vi "main.vi"() -> ()   [LabVIEW 2019]
uses:
  THCD_400/thcd_controls/variable_reference.ctl
  Fridge_Valve/cluster_ref_fridge_valve.ctl
  <vilib>/Instr/_visa.llb/VISA Flush IO Buffer Mask.ctl
  <vilib>/Utility/config.llb/Read Key (String).vi
  subvi_main/Global 1.vi
  <vilib>/Utility/config.llb/Read Key (Path).vi
  <vilib>/Instr/_visa.llb/VISA Configure Serial Port (Instr).vi
  <vilib>/Utility/config.llb/Read Key (Double).vi
  <vilib>/Utility/file.llb/Write Delimited Spreadsheet (DBL).vi
  <vilib>/Utility/config.llb/NI_LVConfig.lvlib
panel:
  out "Status":bool
  in  "Fridge Valve Open Sub Panel":bool
  in  "?":bool
  in  "?":bool
  in  "?":bool
  in  "?":bool
  out "Status":bool
  out "FC1":dbl format="%#_13g"
  out "FC2":dbl format="%#_13g"
  out "FM1":dbl format="%#_13g"
  out "Bypass Valve Opening":dbl format="%_3f"
  out "Main\nFlow":dbl
  out "Vacuum Pressure":dbl
  out "He3 Vapor Pressure":dbl
  out "Writing to file":bool
  out "Status":bool
  out "Boolean 2":bool
  in  "stop":bool
  out "Boolean":bool
  out "He4 Pressure":dbl
  out "Backfill\nPressure\n(Torr)":dbl
  in  "?":bool
  out "Run-Valve Opening":dbl format="%_3f"
  out "Nose Level (%)":dbl(slide) scale=0.0..100.0
  out "?":u8(slide) scale=0.0..100.0
  in  "?":bool
  out "Sep. Pressure":dbl
  out "?":dbl
  in  "kill process":bool
  out "Array 2":bool[](array[boolean])
  out "Error at VISA Read 7":errorcluster
  out "Error at segmenting output 6":errorcluster
  out "Array":bool[](array[boolean])
  out "Error at segmenting output 5":errorcluster
  out "Error at VISA Read 6":errorcluster
  in  "Numeric":dbl
  out "read buffer":string
  in  "STOP VI":bool
  in  "stop 2":bool
  out "error out 5":errorcluster
  out "error out 4":errorcluster
  out "error out 3":errorcluster
  out "error out 2":errorcluster
  out "value 2":path
  out "value":path
  out "error out":errorcluster
  # "CryoControls"
  # "Torr"
  # "Magnet Flow"
  # "Seperator Flow"
  # "Backfill Pressure (Torr)"
  # "Torr"
  # "n/a"
  # "Torr"
  # "MKS 670 / 1000"
  # "MKS 670 /   100"
  # "MKS 670 / He3"
  # "MKS 946"
  # "THCD-400"
  # "%"
  # "%"
  # "Torr"
  # "Fridge Valve"
  # "Fridge Flow"
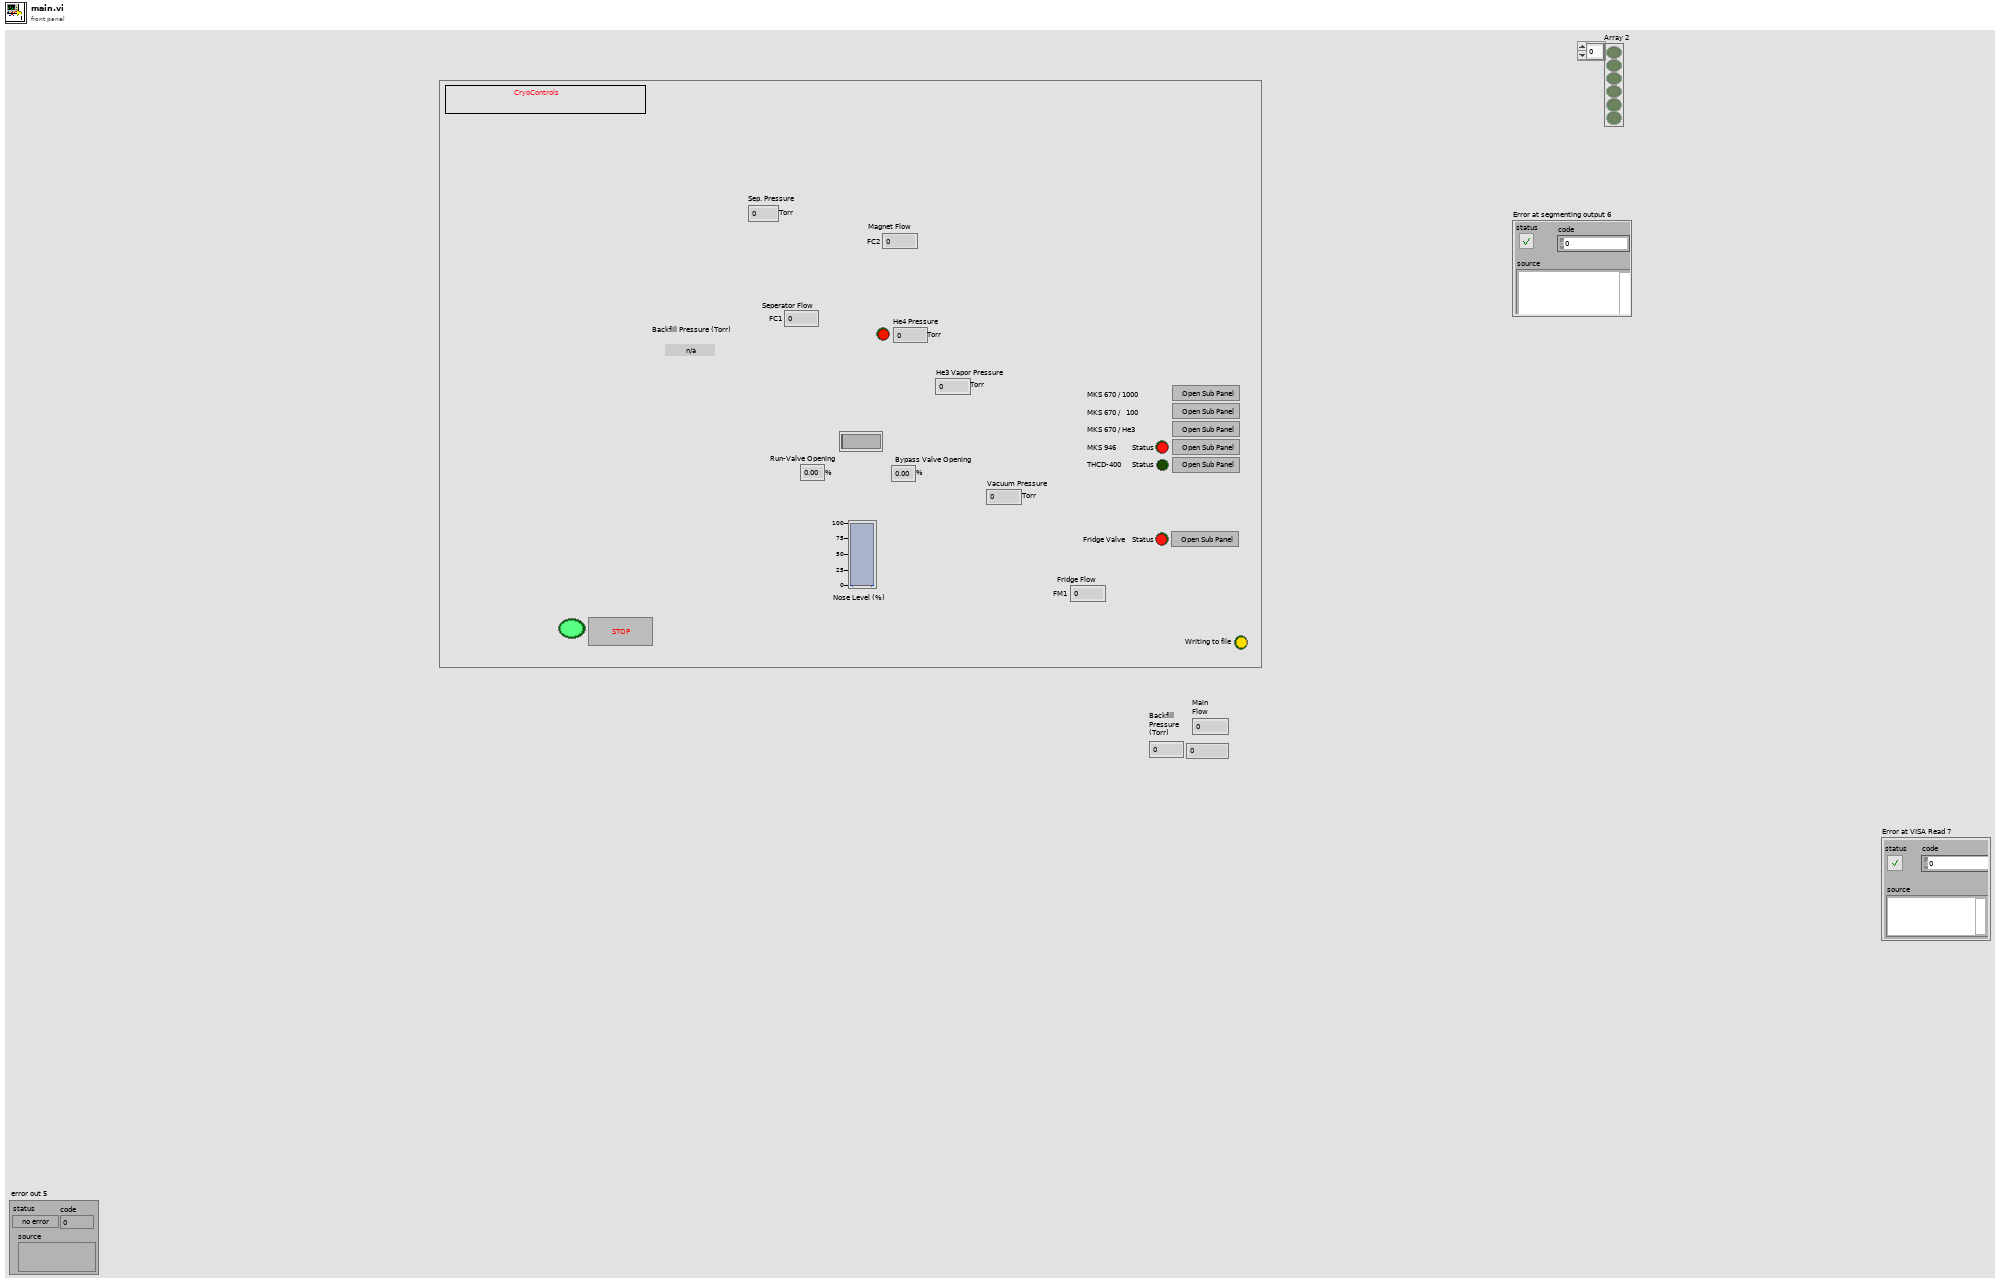
[diagram p1: front panel]
types:
  T1 = typedef "cluster_ref_fridge_valve.ctl" = cluster{"Status":refnum<vi>, "RVO":refnum<vi>, "BVO":refnum<vi>, "He Level":refnum<vi>}
  T2 = typedef "variable_reference.ctl" = cluster{"Status":refnum<vi>, "FM1":refnum<vi>, "FC1":refnum<vi>, "FC2":refnum<vi>}
  T3 = typedef "NI_LVConfig.lvlib/Config Data RefNum.ctl" = refnum<k1>
  T4 = typedef "VISA Flush IO Buffer Mask.ctl" = u16
  T5 = typedef "Semaphore RefNum" = refnum<k1>
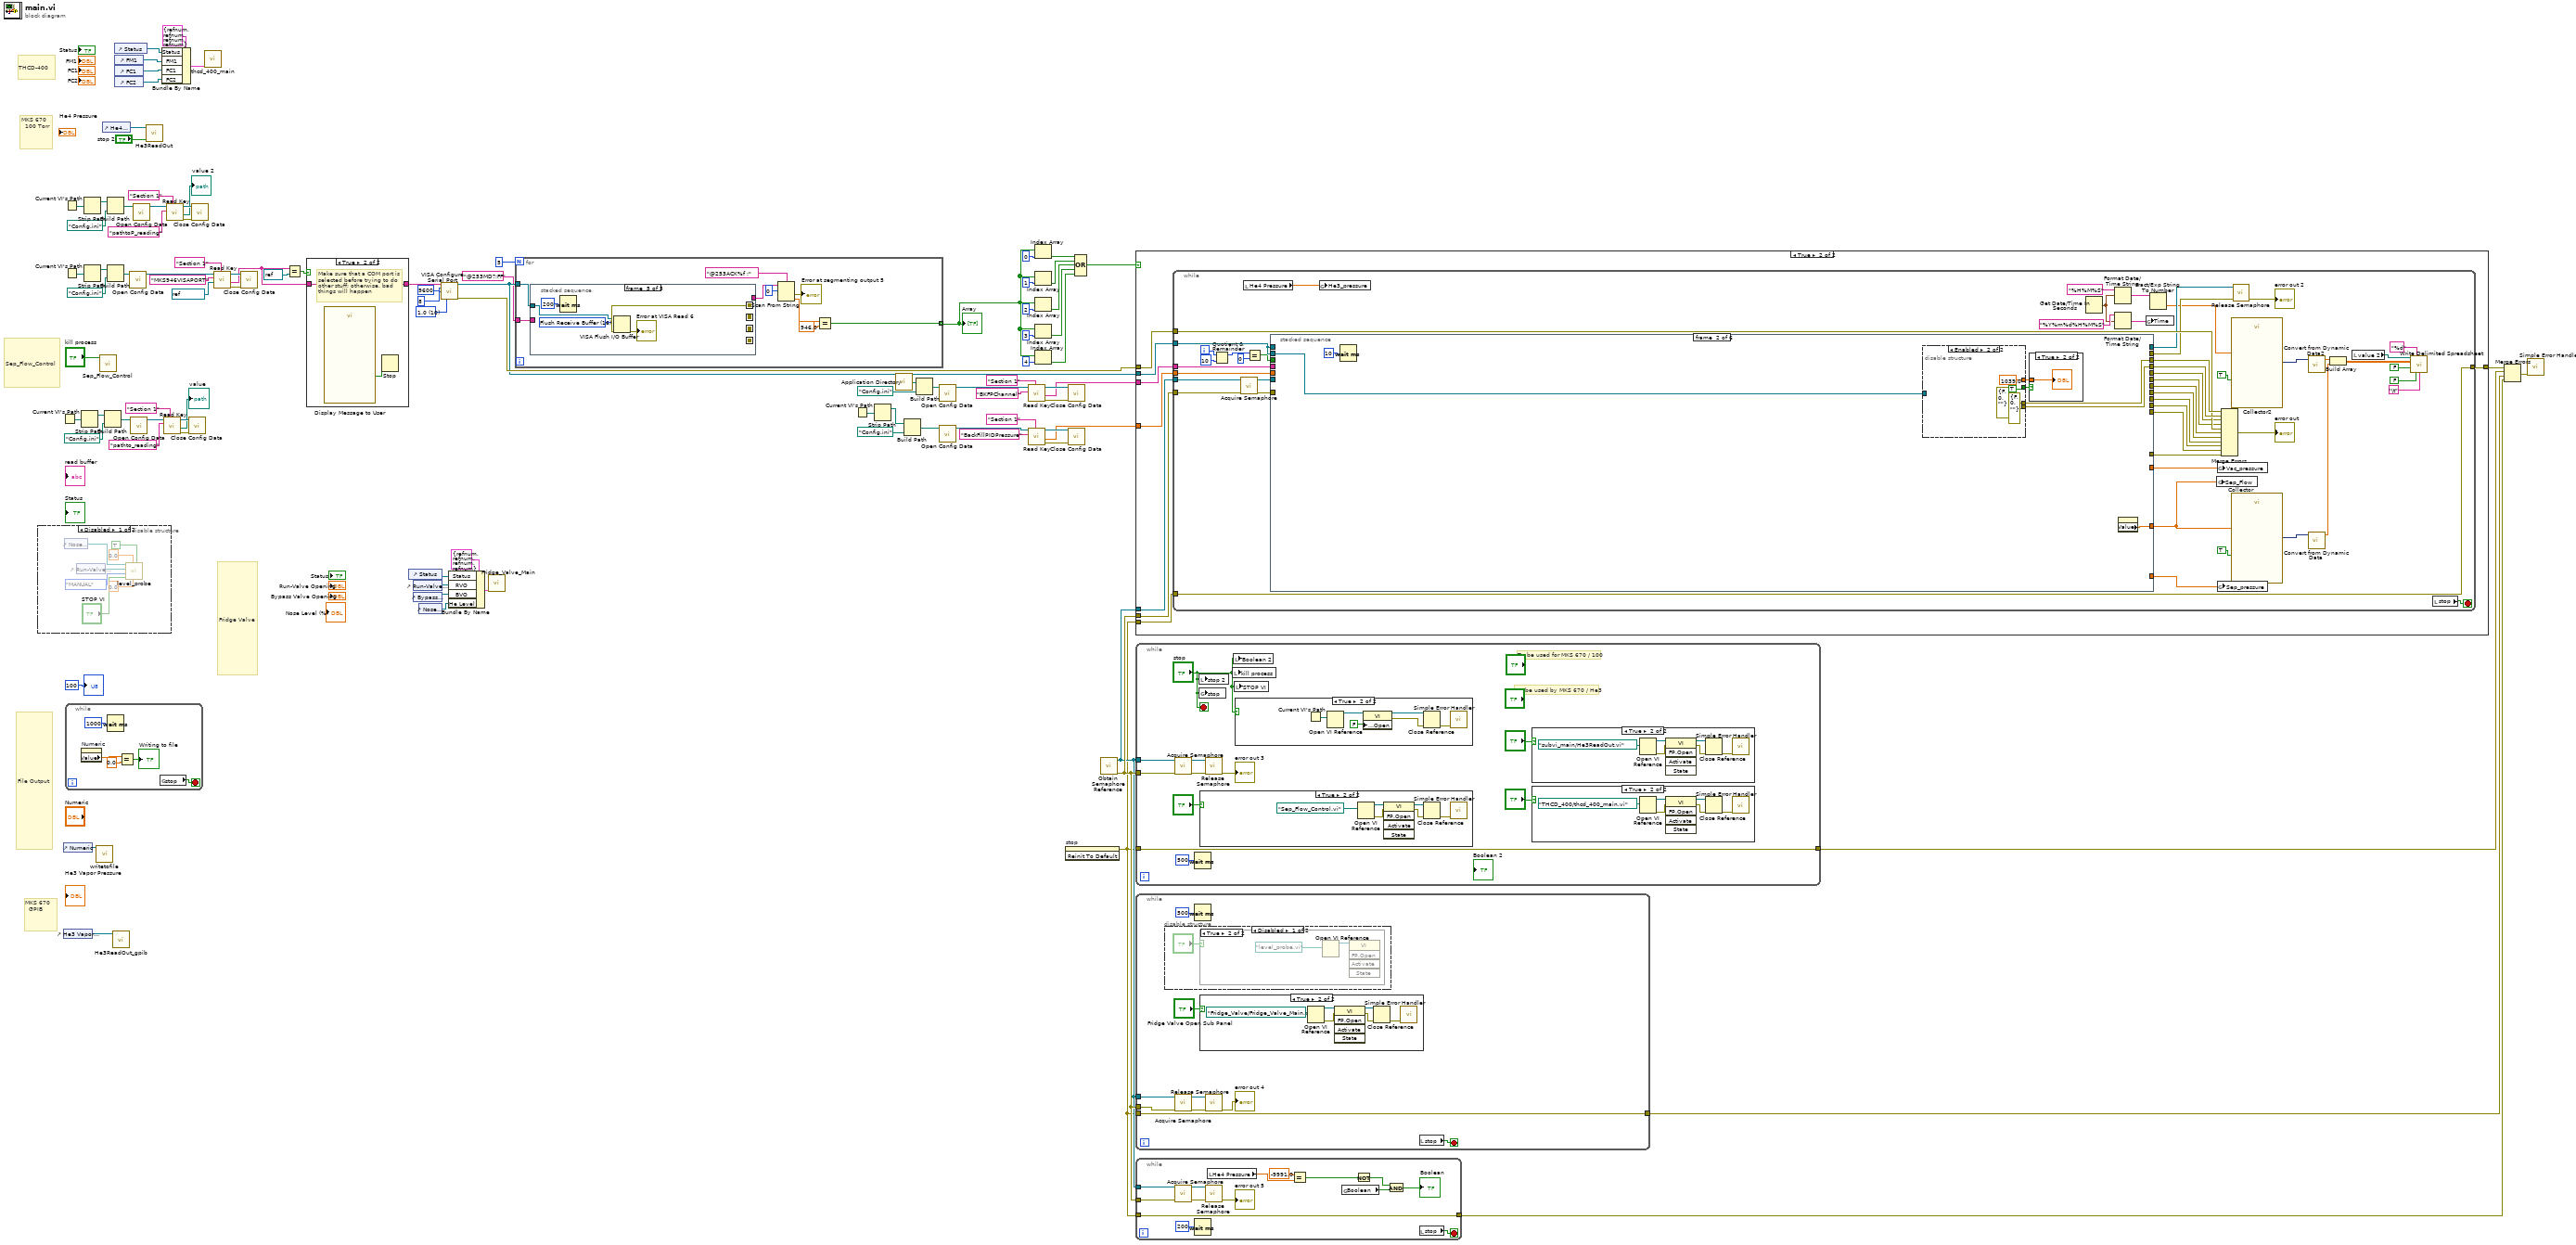
[diagram p0: block diagram]
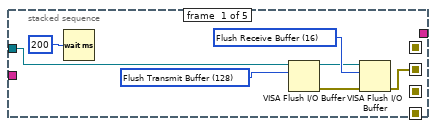
[diagram p3: hidden frame]
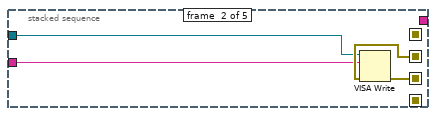
[diagram p4: hidden frame]
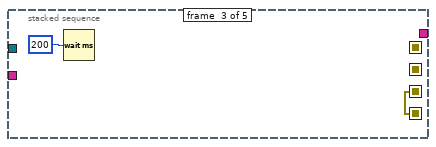
[diagram p5: hidden frame]
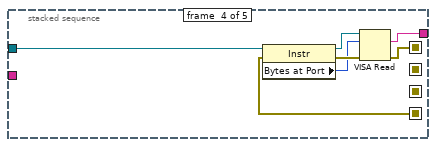
[diagram p6: hidden frame]
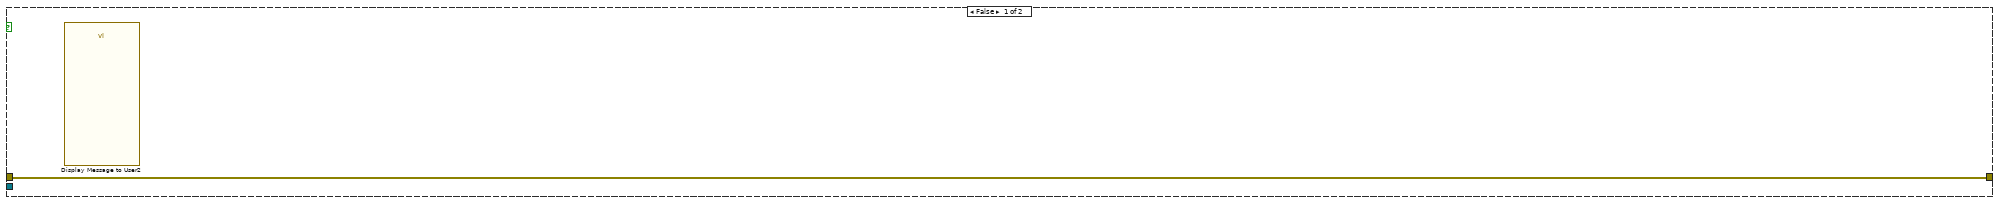
[diagram p7: hidden frame]
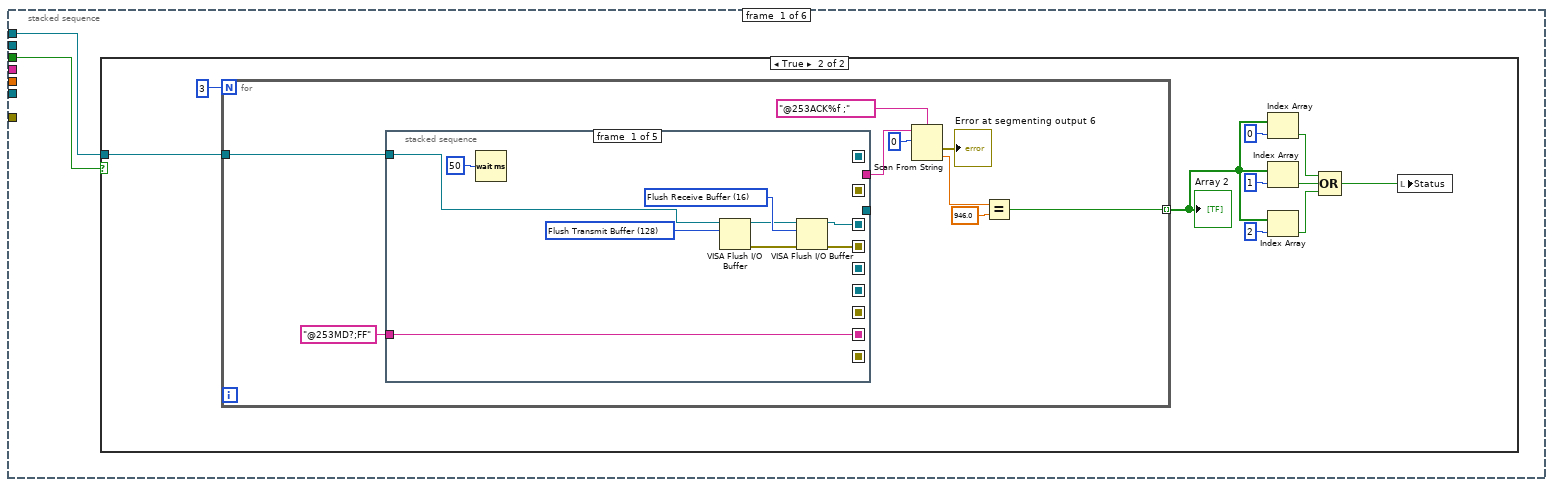
[diagram p8: hidden frame]
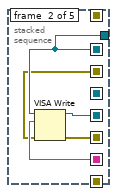
[diagram p10: hidden frame]
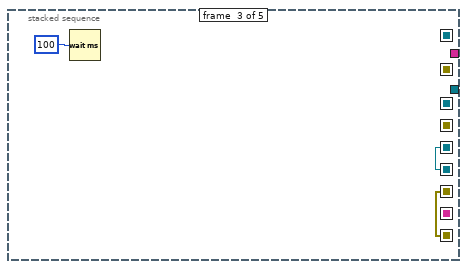
[diagram p11: hidden frame]
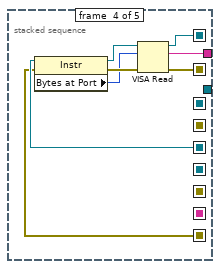
[diagram p12: hidden frame]
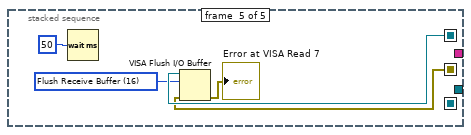
[diagram p13: hidden frame]
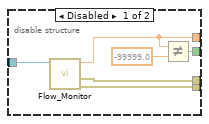
[diagram p14: hidden frame]
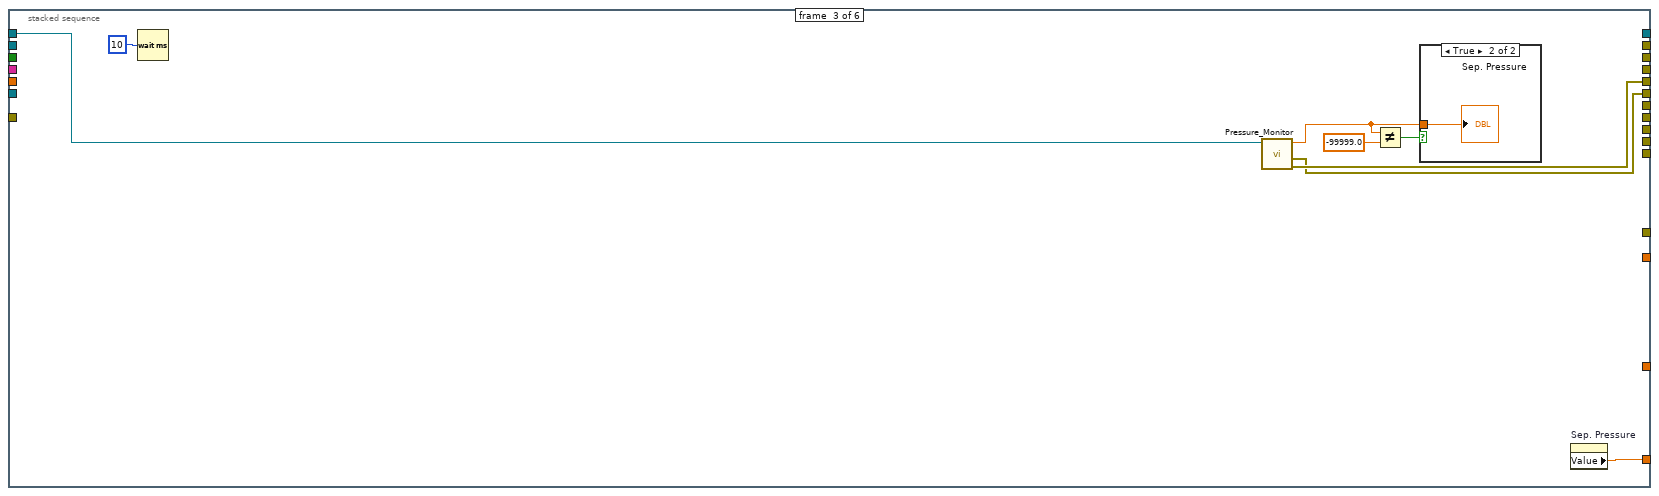
[diagram p16: hidden frame]
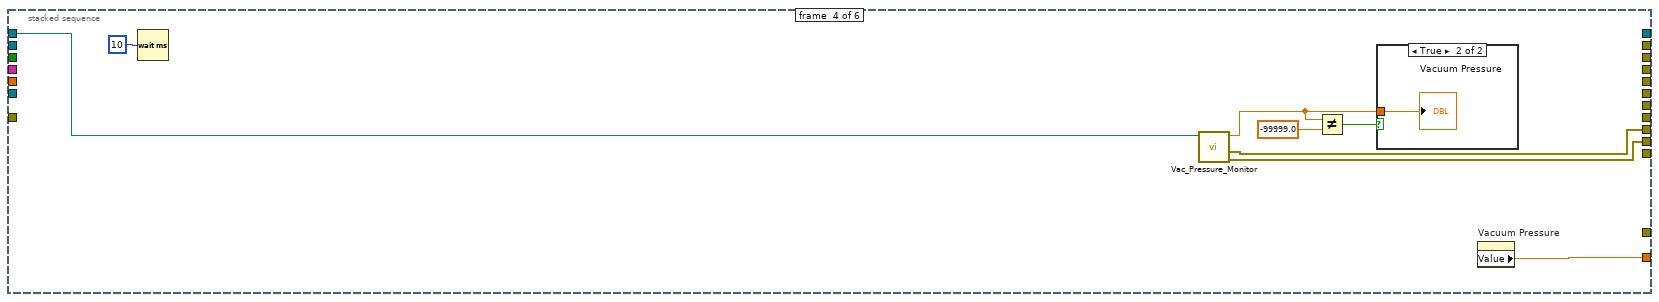
[diagram p18: hidden frame]
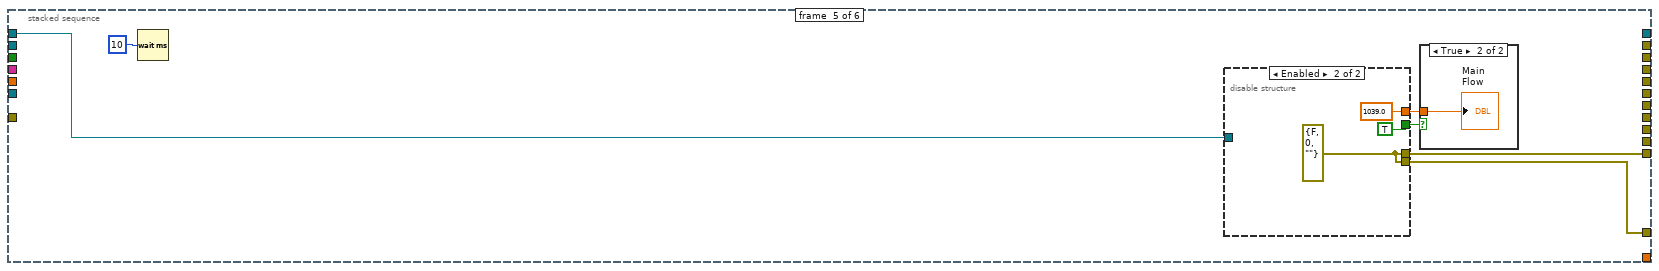
[diagram p20: hidden frame]
diagram:
  w93 = u16 10 items=["1.0"=10, "1.5"=15, "2.0"=20] ("stop bits (10: 1 bit)")
  # "Sep_Flow_Control"
  # "Fridge Valve"
  # "File Output"
  # "MKS 670  \n  GPIB"
  # "MKS 670  \n  100 Torr"
  # "THCD-400"
  n1 = disable-structure shown="Disabled" {
    frame Disabled {
      n2 = control-ref of="Nose Level (%)"() -> (w104:refnum<vi>)
      n3 = control-ref of="Run-Valve Opening"() -> (w105:refnum<vi>)
      n4 = call "level_probe.vi"("Run VI"=TRUE, "Set # of Turns Open (Man)"=0.0, "Target Level (Auto)"=0.0, "stop"="STOP VI", "Mode"=enum32{"AUTOMATIC", "MANUAL"}."MANUAL", "position"=w105, "level"=w104) -> ()  [unwired: 5 in]
    }
    frame Enabled {
    }
  }
  n5 = Current VI's Path() -> (path=w26:path)
  n6 = control-ref of="Numeric"() -> (w46:refnum<vi>)
  n7 = control-ref of="He3 Vapor Pressure"() -> (w14:refnum<vi>)
  n8 = Current VI's Path() -> (path=w30:path)
  n9 = Current VI's Path() -> (path=w28:path)
  n10 = while {
    stop <- w107 stop-if-true
    n11 = property on="Numeric" class="DigNum (strict)"() -> ("Value"=w109:dbl)  [unwired: 2 in, 2 out]
    n12 = Wait (ms)(milliseconds to wait=u32 1000) -> ()  [unwired: 1 out]
    n13 = Equal?(x=w109, y=0.0) -> (x = y?=→"Writing to file":bool)
    n14 = global read "Global 1.vi" "stop"() -> (w107:bool)
  }
  n15 = Strip Path(path=w26) -> (stripped path=w25:path)  [unwired: 1 out]
  n16 = Strip Path(path=w30) -> (stripped path=w29:path)  [unwired: 1 out]
  n17 = Strip Path(path=w28) -> (stripped path=w27:path)  [unwired: 1 out]
  n18 = call "writetofile.vi"("reference"=w46) -> ()  [unwired: 9 in]
  n19 = call "Sep_Flow_Control.vi"("kill process"="kill process") -> ()  [unwired: 11 in]
  n20 = control-ref of="He4 Pressure"() -> (w56:refnum<vi>)
  n21 = Build Path(base path=w25, name or relative path=path "Config.ini" ("default name")) -> (appended path=w67:path)
  n22 = Build Path(base path=w29, name or relative path=path "Config.ini" ("default name")) -> (appended path=w80:path)
  n23 = Build Path(base path=w27, name or relative path=path "Config.ini" ("default name")) -> (appended path=w86:path)
  n24 = call "He3ReadOut_gpib.vi"("reference"=w14) -> ()  [unwired: 11 in]
  n25 = control-ref of="Status"() -> (w11:refnum<vi>)
  n26 = control-ref of="FM1"() -> (w10:refnum<vi>)
  n27 = control-ref of="FC1"() -> (w9:refnum<vi>)
  n28 = control-ref of="FC2"() -> (w8:refnum<vi>)
  n29 = call <vilib>:"Open Config Data.vi"("configuration file path"=w86) -> ("refnum"=w91:T3)  [unwired: 8 in, 2 out]
  n30 = call <vilib>:"Open Config Data.vi"("configuration file path"=w67) -> ("refnum"=w66:T3)  [unwired: 8 in, 2 out]
  n31 = call <vilib>:"Open Config Data.vi"("configuration file path"=w80) -> ("refnum"=w69:T3)  [unwired: 8 in, 2 out]
  n32 = call "He3ReadOut.vi"("reference"=w56, "stop"="stop 2") -> ()  [unwired: 7 in]
  n33 = Bundle By Name(cluster=T2 {"Status"=refnum, "FM1"=refnum, "FC1"=refnum, "FC2"=refnum} ("variable_ref"), "Status"=w11, "FM1"=w10, "FC1"=w9, "FC2"=w8) -> (w7:T2)
  n34 = call-poly <vilib>:"Read Key.vi"("section"="Section 1", "key"="pathto_reading", "refnum"=w66) -> ("error out"=w76:errorcluster, "value"=→"value":path, "refnum out"=w78:T3)  [unwired: 5 in, 1 out]
  n35 = call-poly <vilib>:"Read Key.vi"("section"="Section 1", "key"="pathtoP_reading", "refnum"=w69) -> ("error out"=w71:errorcluster, "value"=→"value 2":path, "refnum out"=w73:T3)  [unwired: 5 in, 1 out]
  n36 = call <vilib>:"Close Config Data.vi"("error in (no error)"=w76, "refnum"=w78) -> ()  [unwired: 8 in, 2 out]
  n37 = call <vilib>:"Close Config Data.vi"("error in (no error)"=w71, "refnum"=w73) -> ()  [unwired: 8 in, 2 out]
  n38 = call "thcd_400_main.vi"("variable_ref"=w7) -> ()  [unwired: 10 in]
  n39 = call-poly <vilib>:"Read Key.vi"("section"="Section 1", "default value"=refnum<visa-resource-name> "COM5" ("VISA resource name"), "key"="MKS946VISAPORT", "refnum"=w91) -> ("error out"=w85:errorcluster, "value"=w83:string, "refnum out"=w89:T3)  [unwired: 4 in, 1 out]
  n40 = call <vilib>:"Close Config Data.vi"("error in (no error)"=w85, "refnum"=w89) -> ()  [unwired: 8 in, 2 out]
  n41 = Equal?(x=w83, y=refnum<visa-resource-name> refnum) -> (x = y?=w97:bool)
  n42 = case shown="True" w97 {
    tunnel: [w111 w112] -> w98
    tunnel: w83 -> [w111 w112]
    frame False {
    }
    frame True {
      # "Make sure that a COM port is\nselected before trying to do\nother stuff; otherwise, bad\nthings will happen"
      n43 = call "Display Message to User"() -> ("Got it, thanks"=w113:bool)  [unwired: 10 in, 1 out]
      n44 = Stop(stop? (T)=w113) -> ()
    }
  }
  n45 = control-ref of="Status"() -> (w6:refnum<vi>)
  n46 = control-ref of="Run-Valve Opening"() -> (w4:refnum<vi>)
  n47 = control-ref of="Bypass Valve Opening"() -> (w3:refnum<vi>)
  n48 = control-ref of="Nose Level (%)"() -> (w1:refnum<vi>)
  n49 = call-poly "VISA Configure Serial Port"("VISA resource name"=w98, "baud rate (9600)"=u32 9600, "data bits (8)"=u16 8, "stop bits (10: 1 bit)"=w93) -> ("VISA resource name out"=w45:refnum<visa-resource-name>, "error out"=w92:errorcluster)  [unwired: 10 in]
  n50 = Bundle By Name(cluster=T1 {"Status"=refnum, "RVO"=refnum, "BVO"=refnum, "He Level"=refnum} ("input cluster"), "Status"=w6, "RVO"=w4, "BVO"=w3, "He Level"=w1) -> (w2:T1)
  n51 = call "Fridge_Valve_Main.vi"("cluster_ref_fridge_valve"=w2) -> ()  [unwired: 11 in]
  n52 = for {
    N: 5 -> [_]
    tunnel: w45 -> [w116]
    tunnel: "@253MD?;FF" ("string") -> [w115]
    tunnel: [w114] -> w31 mode=indexing
    n53 = stacked-sequence {
      seq-local: [w124 _ _ _ _] -> [_ w132 _ _ _]
      seq-local: [_ w133 _ _ _] -> [_ _ w134 _ _]
      seq-local: [_ _ w134 _ _] -> [_ _ _ w139 _]
      seq-local: [_ _ _ w138 _] -> [_ _ _ _ w146]
      tunnel: w115 -> [_ w130 _ _ _]
      tunnel: w116 -> [w125 w131 _ w136 w143]
      tunnel: [_ _ _ w137 _] -> w117
      frame #0 {
        w129 = T4 16 items=["Flush Receive Buffer"=16, "Write Transmit Buffer to Device"=32, "Flush Receive Buffer (No I/O)"=64, "Flush Transmit Buffer"=128] ("Mask")
        w126 = T4 128 items=["Flush Receive Buffer"=16, "Write Transmit Buffer to Device"=32, "Flush Receive Buffer (No I/O)"=64, "Flush Transmit Buffer"=128] ("Mask")
        n54 = Wait (ms)(milliseconds to wait=u32 200) -> ()  [unwired: 1 out]
        n55 = VISA Flush I/O Buffer(VISA resource name=w125, mask (16)=w126) -> (VISA resource name out=w127:refnum<visa-resource-name>, error out=w128:errorcluster)  [unwired: 1 in]
        n56 = VISA Flush I/O Buffer(VISA resource name=w127, mask (16)=w129, error in (no error)=w128) -> (error out=w124:errorcluster)  [unwired: 1 out]
      }
      frame #1 {
        n57 = VISA Write(VISA resource name=w131, write buffer=w130, error in (no error)=w132) -> (error out=w133:errorcluster)  [unwired: 2 out]
      }
      frame #2 {
        n58 = Wait (ms)(milliseconds to wait=u32 200) -> ()  [unwired: 1 out]
      }
      frame #3 {
        n59 = property class="Instr"(reference=w136, error in=w139) -> (reference out=w140:refnum<visa-resource-name>, error out=w142:errorcluster, "Bytes at Port"=w141:u32)
        n60 = VISA Read(VISA resource name=w140, byte count=w141, error in (no error)=w142) -> (read buffer=w137:string, error out=w138:errorcluster)  [unwired: 2 out]
      }
      frame #4 {
        w144 = T4 16 items=["Flush Receive Buffer"=16, "Write Transmit Buffer to Device"=32, "Flush Receive Buffer (No I/O)"=64, "Flush Transmit Buffer"=128] ("Mask")
        n61 = Wait (ms)(milliseconds to wait=u32 200) -> ()  [unwired: 1 out]
        n62 = VISA Flush I/O Buffer(VISA resource name=w143, mask (16)=w144, error in (no error)=w146) -> (error out=→"Error at VISA Read 6":errorcluster)  [unwired: 1 out]
      }
    }
    n63 = Scan From String(format string="@253ACK%f ;", input string=w117, initial scan location=u32 0) -> (error out=→"Error at segmenting output 5":errorcluster, output 1=w119:dbl)  [unwired: 2 in, 2 out]
    n64 = Equal?(x=w119, y=946.0) -> (x = y?=w114:bool)
  }
  "Array" <- w31
  n65 = Current VI's Path() -> (path=w17:path)
  n66 = Strip Path(path=w17) -> (stripped path=w16:path)  [unwired: 1 out]
  n67 = call <vilib>:"Application Directory.vi"() -> ("Application Directory"=w58:path)
  n68 = Build Path(base path=w16, name or relative path=path "Config.ini" ("default name")) -> (appended path=w19:path)
  n69 = Build Path(base path=w58, name or relative path=path "Config.ini" ("default name")) -> (appended path=w60:path)
  n70 = call <vilib>:"Open Config Data.vi"("configuration file path"=w60) -> ("refnum"=w65:T3)  [unwired: 8 in, 2 out]
  n71 = call <vilib>:"Open Config Data.vi"("configuration file path"=w19) -> ("refnum"=w24:T3)  [unwired: 8 in, 2 out]
  n72 = call-poly <vilib>:"Read Key.vi"("section"="Section 1", "key"="BKFPChannel", "refnum"=w65) -> ("error out"=w59:errorcluster, "value"=w57:string, "refnum out"=w63:T3)  [unwired: 5 in, 1 out]
  n73 = call-poly <vilib>:"Read Key.vi"("section"="Section 1", "key"="BackFillPIDPressure", "refnum"=w24) -> ("error out"=w18:errorcluster, "value"=w15:dbl, "refnum out"=w22:T3)  [unwired: 5 in, 1 out]
  n74 = Index Array(array=w31, index=0) -> (element=w36:bool)
  n75 = Index Array(array=w31, index=1) -> (element=w37:bool)
  n76 = Index Array(array=w31, index=2) -> (element=w35:bool)
  n77 = Index Array(array=w31, index=3) -> (element=w34:bool)
  n78 = Index Array(array=w31, index=4) -> (element=w33:bool)
  n79 = invoke on="stop" class="Bool (strict)" method="Reinit To Default"() -> (error out=w49:errorcluster)  [unwired: 3 in, 2 out]
  n80 = call <vilib>:"Close Config Data.vi"("error in (no error)"=w59, "refnum"=w63) -> ()  [unwired: 8 in, 2 out]
  n81 = call <vilib>:"Close Config Data.vi"("error in (no error)"=w18, "refnum"=w22) -> ()  [unwired: 8 in, 2 out]
  n82 = Compound Arithmetic op=OR(w36, w37, w35, w34, w33) -> (w32:bool)
  n83 = call <vilib>:"Obtain Semaphore Reference.vi"() -> ("error out"=w51:errorcluster, "semaphore"=w50:T5)  [unwired: 5 in, 1 out]
  n84 = case shown="True" w32 {
    tunnel: w92 -> [w148 w156]
    tunnel: w57 -> [_ w155]
    tunnel: [w148 w150] -> w55
    tunnel: w51 -> [_ w154]
    tunnel: w50 -> [_ w153]
    tunnel: w49 -> [_ w152]
    tunnel: w45 -> [_ w151]
    tunnel: w15 -> [_ w149]
    frame False {
      n85 = call "Display Message to User2"() -> ()  [unwired: 10 in, 2 out]
    }
    frame True {
      n86 = while {
        tunnel: w151 -> [w190]
        tunnel: w156 -> [w189]
        tunnel: w155 -> [w185]
        tunnel: w153 -> [w182]
        tunnel: w154 -> [w181]
        tunnel: w152 -> [w175]
        tunnel: [w175] -> w150
        tunnel: w149 -> [w163]
        i -> [w173]
        stop <- w174 stop-if-true
        n87 = Quotient & Remainder(x=w173, y=10) -> (x-y*floor(x/y)=w171:i32)  [unwired: 1 out]
        n88 = call <vilib>:"Acquire Semaphore.vi"("error in (no error)"=w181, "semaphore"=w182) -> ("error out"=w179:errorcluster, "semaphore out"=w180:T5)  [unwired: 3 in, 1 out]
        n89 = local read "He4 Pressure"() -> (w166:dbl)
        n90 = Equal?(x=w171, y=0) -> (x = y?=w169:bool)
        n91 = stacked-sequence {
          tunnel: w190 -> [_ w262 _ _ _ _]
          tunnel: w190 -> [w209 _ w280 w289 w297 w314]
          tunnel: w180 -> [_ _ _ _ _ w313]
          tunnel: w179 -> [_ _ _ _ _ w311]
          tunnel: w169 -> [w208 _ _ _ _ _]
          tunnel: w185 -> [_ _ _ _ _ w315]
          tunnel: w163 -> [_ _ _ _ _ w312]
          tunnel: [_ w259 _ _ _ _] -> w207
          tunnel: [_ w260 _ _ _ _] -> w206
          tunnel: [_ w261 _ _ _ _] -> w167
          tunnel: [_ _ w279 _ _ _] -> w164
          tunnel: [_ _ w278 _ _ _] -> w184
          tunnel: [_ _ w277 _ _ _] -> w183
          tunnel: [_ _ _ w288 _ _] -> w161
          tunnel: [_ _ _ w287 _ _] -> w160
          tunnel: [_ _ _ w286 _ _] -> w159
          tunnel: [_ _ _ _ _ w321] -> w187
          tunnel: [_ _ _ _ _ w320] -> w186
          tunnel: [_ _ _ _ _ w313] -> w178
          tunnel: [_ _ _ _ _ w311] -> w177
          tunnel: [_ _ _ _ w296 _] -> w158
          tunnel: [_ _ _ _ w295 _] -> w157
          frame #0 {
            n92 = case shown="True" w208 {
              tunnel: w209 -> [_ w210]
              frame False {
              }
              frame True {
                n93 = for {
                  N: 3 -> [_]
                  tunnel: w210 -> [w222]
                  tunnel: [w221] -> w219 mode=indexing
                  n94 = stacked-sequence {
                    seq-local: [w237 _ _ _ _] -> [_ w242 _ _ _]
                    seq-local: [w231 _ _ _ _] -> [_ w239 _ _ _]
                    seq-local: [w230 _ _ _ _] -> [_ w238 _ _ _]
                    seq-local: [_ w241 _ _ _] -> [_ _ w244 _ _]
                    seq-local: [_ w240 _ _ _] -> [_ _ w243 _ _]
                    seq-local: [_ _ w244 _ _] -> [_ _ _ w250 _]
                    seq-local: [_ _ w243 _ _] -> [_ _ _ w249 _]
                    seq-local: [_ _ _ w248 _] -> [_ _ _ _ w257]
                    seq-local: [_ _ _ w247 _] -> [_ _ _ _ w256]
                    tunnel: "@253MD?;FF" ("string") -> [w237 _ _ _ _]
                    tunnel: w222 -> [w232 _ _ _ _]
                    tunnel: [_ w239 _ _ _] -> _
                    tunnel: [_ _ _ w246 _] -> w223
                    frame #0 {
                      w236 = T4 16 items=["Flush Receive Buffer"=16, "Write Transmit Buffer to Device"=32, "Flush Receive Buffer (No I/O)"=64, "Flush Transmit Buffer"=128] ("Mask")
                      w233 = T4 128 items=["Flush Receive Buffer"=16, "Write Transmit Buffer to Device"=32, "Flush Receive Buffer (No I/O)"=64, "Flush Transmit Buffer"=128] ("Mask")
                      n95 = Wait (ms)(milliseconds to wait=u32 50) -> ()  [unwired: 1 out]
                      n96 = VISA Flush I/O Buffer(VISA resource name=w232, mask (16)=w233) -> (VISA resource name out=w234:refnum<visa-resource-name>, error out=w235:errorcluster)  [unwired: 1 in]
                      n97 = VISA Flush I/O Buffer(VISA resource name=w234, mask (16)=w236, error in (no error)=w235) -> (VISA resource name out=w231:refnum<visa-resource-name>, error out=w230:errorcluster)
                    }
                    frame #1 {
                      n98 = VISA Write(VISA resource name=w239, write buffer=w242, error in (no error)=w238) -> (VISA resource name out=w241:refnum<visa-resource-name>, error out=w240:errorcluster)  [unwired: 1 out]
                    }
                    frame #2 {
                      n99 = Wait (ms)(milliseconds to wait=u32 100) -> ()  [unwired: 1 out]
                    }
                    frame #3 {
                      n100 = property class="Instr"(reference=w250, error in=w249) -> (reference out=w251:refnum<visa-resource-name>, error out=w253:errorcluster, "Bytes at Port"=w252:u32)
                      n101 = VISA Read(VISA resource name=w251, byte count=w252, error in (no error)=w253) -> (VISA resource name out=w248:refnum<visa-resource-name>, read buffer=w246:string, error out=w247:errorcluster)  [unwired: 1 out]
                    }
                    frame #4 {
                      w254 = T4 16 items=["Flush Receive Buffer"=16, "Write Transmit Buffer to Device"=32, "Flush Receive Buffer (No I/O)"=64, "Flush Transmit Buffer"=128] ("Mask")
                      n102 = Wait (ms)(milliseconds to wait=u32 50) -> ()  [unwired: 1 out]
                      n103 = VISA Flush I/O Buffer(VISA resource name=w257, mask (16)=w254, error in (no error)=w256) -> (error out=→"Error at VISA Read 7":errorcluster)  [unwired: 1 out]
                    }
                  }
                  n104 = Scan From String(format string="@253ACK%f ;", input string=w223, initial scan location=u32 0) -> (error out=→"Error at segmenting output 6":errorcluster, output 1=w225:dbl)  [unwired: 2 in, 2 out]
                  n105 = Equal?(x=w225, y=946.0) -> (x = y?=w221:bool)
                }
                "Array 2" <- w219
                n106 = Index Array(array=w219, index=0) -> (element=w217:bool)
                n107 = Index Array(array=w219, index=1) -> (element=w216:bool)
                n108 = Index Array(array=w219, index=2) -> (element=w218:bool)
                n109 = Compound Arithmetic op=OR(w217, w216, w218) -> (w211:bool)
                n110 = local write "Status"(w211) -> ()
              }
            }
          }
          frame #1 {
            n111 = Wait (ms)(milliseconds to wait=u32 10) -> ()  [unwired: 1 out]
            n112 = disable-structure shown="Enabled" {
              disable-tunnel: [w270 TRUE] -> w265
              disable-tunnel: [w269 1039.0 ("Flow readout")] -> w263
              disable-tunnel: w262 -> [w268 _]
              disable-tunnel: [w267 errorcluster {"status"=FALSE, "code"=0, "source"=""} ("Error at segmenting output")] -> w260
              disable-tunnel: [w266 errorcluster {"status"=FALSE, "code"=0, "source"=""} ("Error at VISA Read")] -> w259
              frame Disabled {
                n113 = call "Flow_Monitor.vi"("VISA resource name"=w268) -> ("Error at segmenting output"=w267:errorcluster, "Error at VISA Read"=w266:errorcluster, "Flow readout"=w269:dbl)  [unwired: 8 in]
                n114 = Not Equal?(x=w269, y=-99999.0) -> (x != y?=w270:bool)
              }
              frame Enabled {
              }
            }
            n115 = case shown="True" w265 {
              tunnel: w263 -> [_ w276]
              frame False {
              }
              frame True {
                "?" <- w276
              }
            }
            n116 = property class="DigNum (strict)"() -> ("Value"=w261:dbl)  [unwired: 2 in, 2 out]
          }
          frame #2 {
            n117 = Wait (ms)(milliseconds to wait=u32 10) -> ()  [unwired: 1 out]
            n118 = call "Pressure_Monitor.vi"("VISA resource name"=w280) -> ("Error at segmenting output"=w278:errorcluster, "Error at VISA Read"=w277:errorcluster, "Flow readout"=w282:dbl)  [unwired: 8 in]
            n119 = Not Equal?(x=w282, y=-99999.0) -> (x != y?=w284:bool)
            n120 = case shown="True" w284 {
              tunnel: w282 -> [_ w285]
              frame False {
              }
              frame True {
                "Sep. Pressure" <- w285
              }
            }
            n121 = property on="Sep. Pressure" class="DigNum (strict)"() -> ("Value"=w279:dbl)  [unwired: 2 in, 2 out]
          }
          frame #3 {
            n122 = Wait (ms)(milliseconds to wait=u32 10) -> ()  [unwired: 1 out]
            n123 = call "Vac_Pressure_Monitor.vi"("VISA resource name"=w289) -> ("Error at segmenting output"=w287:errorcluster, "Error at VISA Read"=w288:errorcluster, "Flow readout"=w290:dbl)  [unwired: 8 in]
            n124 = Not Equal?(x=w290, y=-99999.0) -> (x != y?=w292:bool)
            n125 = case shown="True" w292 {
              tunnel: w290 -> [_ w294]
              frame False {
              }
              frame True {
                "Vacuum Pressure" <- w294
              }
            }
            n126 = property on="Vacuum Pressure" class="DigNum (strict)"() -> ("Value"=w286:dbl)  [unwired: 2 in, 2 out]
          }
          frame #4 {
            n127 = Wait (ms)(milliseconds to wait=u32 10) -> ()  [unwired: 1 out]
            n128 = disable-structure shown="Enabled" {
              disable-tunnel: [w306 1039.0 ("Flow readout")] -> w300
              disable-tunnel: [w304 TRUE] -> w299
              disable-tunnel: w297 -> [w303 _]
              disable-tunnel: [w302 w307] -> w296
              disable-tunnel: [w301 w307] -> w295
              frame Disabled {
                n129 = call "MainFlow_Monitor.vi"("VISA resource name"=w303) -> ("Error at segmenting output"=w301:errorcluster, "Error at VISA Read"=w302:errorcluster, "Flow readout"=w306:dbl)  [unwired: 8 in]
                n130 = Not Equal?(x=w306, y=-99999.0) -> (x != y?=w304:bool)
              }
              frame Enabled {
                w307 = errorcluster {"status"=FALSE, "code"=0, "source"=""} ("Error at VISA Read")
              }
            }
            n131 = case shown="True" w299 {
              tunnel: w300 -> [_ w310]
              frame False {
              }
              frame True {
                "Main\nFlow" <- w310
              }
            }
          }
          frame #5 {
            n132 = Wait (ms)(milliseconds to wait=u32 10) -> ()  [unwired: 1 out]
            n133 = disable-structure shown="Enabled" {
              disable-tunnel: [w328 w343] -> w321
              disable-tunnel: [w327 w343] -> w320
              disable-tunnel: [w325 1039.0] -> w317
              disable-tunnel: w315 -> [w324 _]
              disable-tunnel: w314 -> [w323 _]
              disable-tunnel: w312 -> [w322 _]
              frame Disabled {
                n134 = call "Pressure_Monitor_bkfl.vi"("VISA resource name"=w323) -> ("Error at segmenting output"=w327:errorcluster, "Error at VISA Read"=w328:errorcluster, "Flow readout"=w325:dbl)  [unwired: 8 in]
                n135 = Greater?(x=w322, y=w325) -> (0:w326:bool)
                n136 = case shown="True" w326 {
                  tunnel: w324 -> [w331 w338]
                  tunnel: w323 -> [w330 w337]
                  frame False {
                    n137 = Concatenate Strings("@253QMD", w331, "!Open;FF") -> (w332:string)
                    n138 = VISA Write(VISA resource name=w330, write buffer=w332) -> (VISA resource name out=w329:refnum<visa-resource-name>)  [unwired: 1 in, 2 out]
                    n139 = VISA Clear(VISA resource name=w329) -> ()  [unwired: 1 in, 2 out]
                  }
                  frame True {
                    n140 = Concatenate Strings("@253QMD", w338, "!Close;FF") -> (w339:string)
                    n141 = VISA Write(VISA resource name=w337, write buffer=w339) -> (VISA resource name out=w335:refnum<visa-resource-name>, error out=w336:errorcluster)  [unwired: 1 in, 1 out]
                    n142 = VISA Clear(VISA resource name=w335, error in (no error)=w336) -> ()  [unwired: 2 out]
                  }
                }
              }
              frame Enabled {
                w343 = errorcluster {"status"=FALSE, "code"=0, "source"=""} ("Error at VISA Read")
              }
            }
            n143 = Not Equal?(x=w317, y=-99999.0) -> (x != y?=w319:bool)
            n144 = case shown="True" w319 {
              tunnel: w317 -> [_ w344]
              frame False {
              }
              frame True {
                "Backfill\nPressure\n(Torr)" <- w344
              }
            }
          }
        }
        n145 = global write "Global 1.vi" "He3_pressure"(w166) -> ()
        n146 = Get Date/Time In Seconds() -> (seconds since 1Jan1904=w193:timestamp)
        n147 = Format Date/Time String(time format string (%c)="%H%M%S", seconds (now)=w193) -> (date/time string=w191:string)  [unwired: 1 in]
        n148 = Format Date/Time String(time format string (%c)="%Y%m%d%H%M%S", seconds (now)=w193) -> (date/time string=w165:string)  [unwired: 1 in]
        n149 = global write "Global 1.vi" "Time"(w165) -> ()
        n150 = Fract/Exp String To Number(string=w191) -> (number=w168:dbl)  [unwired: 3 in, 1 out]
        n151 = global write "Global 1.vi" "Sep_Flow"(w167) -> ()
        n152 = global write "Global 1.vi" "Vac_pressure"(w159) -> ()
        n153 = global write "Global 1.vi" "Sep_pressure"(w164) -> ()
        n154 = Merge Errors(w207, w206, w184, w183, w189, w187, w186, w161, w160, w158, w157) -> (→"error out":errorcluster)
        n155 = call "Collector2"("Enable"=TRUE, "Signals"=w168) -> ("Collected Signals"=w197:dynamicdata)  [unwired: 8 in, 1 out]
        n156 = call "Collector"("Enable"=TRUE, "Signals"=w167) -> ("Collected Signals"=w200:dynamicdata)  [unwired: 8 in, 1 out]
        n157 = call <vilib>:"Release Semaphore.vi"("error in (no error)"=w177, "semaphore"=w178) -> ("error out"=→"error out 2":errorcluster)  [unwired: 4 in, 1 out]
        n158 = call "Convert from Dynamic Data2"("Dynamic Data Type"=w197) -> ("Array"=w194:dbl[])  [unwired: 3 in]
        n159 = call "Convert from Dynamic Data"("Dynamic Data Type"=w200) -> ("Array"=w195:dbl[])  [unwired: 3 in]
        n160 = Build Array(w194, w195) -> (w196:dbl[][])
        n161 = local read "value 2"() -> (w162:path)
        n162 = call-poly <vilib>:"Write Delimited Spreadsheet.vi"("file path (dialog if empty)"=w162, "format (%.3f)"="%d", "2D data"=w196, "append to file? (new file:F)"=FALSE, "transpose? (no:F)"=FALSE ("transpose? (F)"), "delimiter (\\t)"="\t" ("delimiter (\\t)")) -> ()  [unwired: 8 in, 2 out]
        n163 = local read "stop"() -> (w174:bool)
      }
    }
  }
  n164 = while {
    tunnel: w50 -> [w354]
    tunnel: w51 -> [w349]
    tunnel: [w350] -> w47
    tunnel: w49 -> [w350]
    stop <- "stop" stop-if-true
    # "To be used by MKS 670 / He3"
    # "To be used for MKS 670 / 100"
    n165 = call <vilib>:"Acquire Semaphore.vi"("error in (no error)"=w349, "semaphore"=w354) -> ("error out"=w352:errorcluster, "semaphore out"=w353:T5)  [unwired: 3 in, 1 out]
    n166 = Wait (ms)(milliseconds to wait=u32 500) -> ()  [unwired: 1 out]
    n167 = local write "stop 2"("stop") -> ()
    n168 = global write "Global 1.vi" "stop"("stop") -> ()
    n169 = case shown="True" "?" {
      frame False {
      }
      frame True {
        n170 = Open VI Reference(vi path=path "Sep_Flow_Control.vi") -> (vi reference=w378:refnum<vi>, error out=w377:errorcluster)  [unwired: 5 in]
        n171 = invoke class="VI" method="FP.Open"(reference=w378, error in=w377) -> (reference out=w375:refnum<vi>, error out=w374:errorcluster)  [unwired: 3 in, 3 out]
        n172 = Close Reference(reference=w375, error in (no error)=w374) -> (error out=w376:errorcluster)
        n173 = call <vilib>:"Simple Error Handler.vi"("error in (no error)"=w376) -> ()  [unwired: 4 in, 5 out]
      }
    }
    n174 = call <vilib>:"Release Semaphore.vi"("error in (no error)"=w352, "semaphore"=w353) -> ("error out"=→"error out 3":errorcluster)  [unwired: 4 in, 1 out]
    n175 = local write "kill process"("stop") -> ()
    n176 = local write "Boolean 2"("stop") -> ()
    n177 = local write "STOP VI"("stop") -> ()
    n178 = case shown="True" "stop" {
      frame False {
      }
      frame True {
        n179 = Current VI's Path() -> (path=w373:path)
        n180 = Open VI Reference(vi path=w373) -> (vi reference=w372:refnum<vi>)  [unwired: 5 in, 1 out]
        n181 = property class="VI"(reference=w372, "Front Panel Window:Open"=FALSE) -> (reference out=w369:refnum<vi>, error out=w368:errorcluster)  [unwired: 1 in]
        n182 = Close Reference(reference=w369, error in (no error)=w368) -> (error out=w370:errorcluster)
        n183 = call <vilib>:"Simple Error Handler.vi"("error in (no error)"=w370) -> ()  [unwired: 4 in, 5 out]
      }
    }
    n184 = case shown="True" "?" {
      frame False {
      }
      frame True {
        n185 = Open VI Reference(vi path=path "subvi_main/He3ReadOut.vi") -> (vi reference=w360:refnum<vi>, error out=w359:errorcluster)  [unwired: 5 in]
        n186 = invoke class="VI" method="FP.Open"(reference=w360, error in=w359) -> (reference out=w357:refnum<vi>, error out=w356:errorcluster)  [unwired: 3 in, 3 out]
        n187 = Close Reference(reference=w357, error in (no error)=w356) -> (error out=w358:errorcluster)
        n188 = call <vilib>:"Simple Error Handler.vi"("error in (no error)"=w358) -> ()  [unwired: 4 in, 5 out]
      }
    }
    n189 = case shown="True" "?" {
      frame False {
      }
      frame True {
        n190 = Open VI Reference(vi path=path "THCD_400/thcd_400_main.vi") -> (vi reference=w366:refnum<vi>, error out=w365:errorcluster)  [unwired: 5 in]
        n191 = invoke class="VI" method="FP.Open"(reference=w366, error in=w365) -> (reference out=w363:refnum<vi>, error out=w362:errorcluster)  [unwired: 3 in, 3 out]
        n192 = Close Reference(reference=w363, error in (no error)=w362) -> (error out=w364:errorcluster)
        n193 = call <vilib>:"Simple Error Handler.vi"("error in (no error)"=w364) -> ()  [unwired: 4 in, 5 out]
      }
    }
  }
  n194 = while {
    tunnel: w50 -> [w387]
    tunnel: w51 -> [w386]
    tunnel: w49 -> [w382]
    tunnel: [w382] -> w54
    stop <- w381 stop-if-true
    n195 = disable-structure shown="Disabled" {
      frame Disabled {
        n196 = case shown="True" "?" {
          frame False {
          }
          frame True {
            n197 = Open VI Reference(vi path=path "level_probe.vi") -> (vi reference=w390:refnum<vi>)  [unwired: 5 in, 1 out]
            n198 = invoke class="VI" method="FP.Open"(reference=w390) -> ()  [unwired: 4 in, 5 out]
          }
        }
      }
      frame Enabled {
      }
    }
    n199 = call <vilib>:"Acquire Semaphore.vi"("error in (no error)"=w386, "semaphore"=w387) -> ("error out"=w384:errorcluster, "semaphore out"=w385:T5)  [unwired: 3 in, 1 out]
    n200 = Wait (ms)(milliseconds to wait=u32 500) -> ()  [unwired: 1 out]
    n201 = case shown="True" "Fridge Valve Open Sub Panel" {
      frame False {
      }
      frame True {
        n202 = Open VI Reference(vi path=path "Fridge_Valve/Fridge_Valve_Main.vi") -> (vi reference=w396:refnum<vi>, error out=w395:errorcluster)  [unwired: 5 in]
        n203 = invoke class="VI" method="FP.Open"(reference=w396, error in=w395) -> (reference out=w393:refnum<vi>, error out=w392:errorcluster)  [unwired: 3 in, 3 out]
        n204 = Close Reference(reference=w393, error in (no error)=w392) -> (error out=w394:errorcluster)
        n205 = call <vilib>:"Simple Error Handler.vi"("error in (no error)"=w394) -> ()  [unwired: 4 in, 5 out]
      }
    }
    n206 = call <vilib>:"Release Semaphore.vi"("error in (no error)"=w384, "semaphore"=w385) -> ("error out"=→"error out 4":errorcluster)  [unwired: 4 in, 1 out]
    n207 = local read "stop"() -> (w381:bool)
  }
  n208 = while {
    tunnel: w49 -> [w409]
    tunnel: [w409] -> w52
    tunnel: w51 -> [w405]
    tunnel: w50 -> [w404]
    stop <- w403 stop-if-true
    n209 = call <vilib>:"Acquire Semaphore.vi"("error in (no error)"=w405, "semaphore"=w404) -> ("error out"=w407:errorcluster, "semaphore out"=w408:T5)  [unwired: 3 in, 1 out]
    n210 = Wait (ms)(milliseconds to wait=u32 200) -> ()  [unwired: 1 out]
    n211 = call <vilib>:"Release Semaphore.vi"("error in (no error)"=w407, "semaphore"=w408) -> ("error out"=→"error out 5":errorcluster)  [unwired: 4 in, 1 out]
    n212 = local read "He4 Pressure"() -> (w402:dbl)
    n213 = Equal?(x=-9991.0, y=w402) -> (x = y?=w399:bool)
    n214 = global read "Global 1.vi" "Boolean"() -> (w401:bool)
    n215 = Not(x=w399) -> (.not. x?=w398:bool)
    n216 = And(x=w398, y=w401) -> (x .and. y?=→"Boolean":bool)
    n217 = local read "stop"() -> (w403:bool)
  }
  n218 = Merge Errors(w55, w47, w54, w52) -> (w53:errorcluster)
  n219 = call <vilib>:"Simple Error Handler.vi"("error in (no error)"=w53) -> ()  [unwired: 4 in, 5 out]
  "?" <- u8 100
